vi "Set VI Icon.vi"(8 "error in (no error)":errorcluster caption="错误输入（无错误）", 10 "路径":path, 11 "VI引用句柄":refnum<vi>) -> (0 "error out":errorcluster caption="错误输出", 2 "OldHandle":u32, 3 "ImageHandle":u32)   [LabVIEW 2013]
uses:
  USER32.DLL
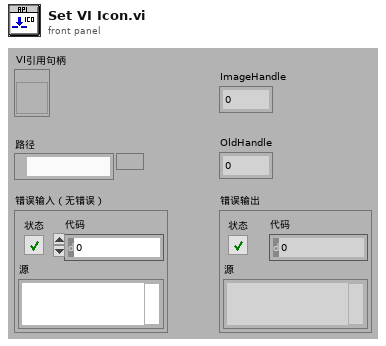
[diagram p1: front panel]
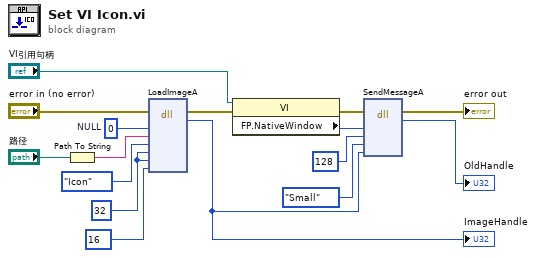
[diagram p0: block diagram]
diagram:
  w15 = u32 32 ("cxDesired")
  w16 = u32 0  # NULL
  n1 = Path To String(path="路径") -> (string=w13:string)
  n2 = dll-call lib="user32.dll" fn="LoadImageA" label="LoadImage"(error in="error in (no error)", "HINSTANCE"=w16, "LPCTSTR"=w13, "uType"=enum16{"Bitmap", "Icon", "Cursor"}."Icon", "cxDesired"=w15, "cyDesired"=w15, "fuLoad"=16) -> (error out=w3:errorcluster, "ImageHandle"=w8:u32)  [unwired: 8 in, 1 out]
  "ImageHandle" <- w8
  n3 = property class="VI"(reference="VI引用句柄", error in=w3) -> (error out=w2:errorcluster, "FP.NativeWindow"=w6:u64)  [unwired: 1 out]
  n4 = dll-call lib="user32.dll" fn="SendMessageA" label="SendMessage"(error in=w2, "hWnd"=w6, "uMsg"=u32 128 ("dimension size"), "wParam"=enum16{"Small", "Big"}."Small", "lParam"=w8) -> (error out=→"error out":errorcluster, "OldHandle"=→"OldHandle":u32)  [unwired: 6 in, 1 out]
